vi "GetType.vi"(8 "error in (no error)":errorcluster, 11 "Disable All Data Markers [DM] Msg":refnum<class "Disable All Data Markers [DM] Msg.lvclass">) -> (0 "error out":errorcluster, 2 "Data Sample":variant, 3 "Disable All Data Markers [DM] Msg":refnum<class "Disable All Data Markers [DM] Msg.lvclass">)   [LabVIEW 2016, in "CS++Fgen.lvlib" / "Disable All Data Markers [DM] Msg.lvclass"]
doc: "This VI delivers a sample of the data type format the message expects."
uses:
  Disable All Data Markers [DM] Msg.lvclass
  Disable All Data Markers [DM] Msg.lvclass/Disable All Data Markers [DM] Msg.ctl
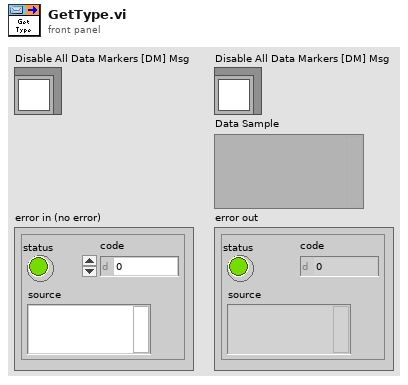
[diagram p1: front panel]
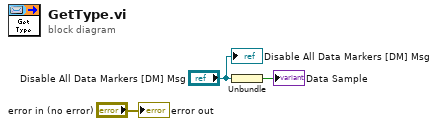
[diagram p0: block diagram]
diagram:
  n1 = Unbundle("Disable All Data Markers [DM] Msg") -> (→"Data Sample":bool)
  "error out" <- "error in (no error)"
  "Disable All Data Markers [DM] Msg" <- "Disable All Data Markers [DM] Msg"
